vi "All Lamps OFF.vi"(7 "L1 Prime":bool=TRUE, 8 "error in (no error)":errorcluster) -> (0 "error out":T1)   [LabVIEW 2018]
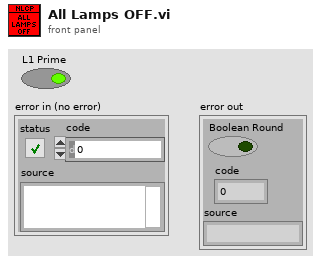
[diagram p1: front panel]
types:
  T1 = cluster{"Boolean Round":bool, "code":i32, "source":string}
  T2 = enum16{"Lamp A1", "Lamp B1", "Lamp C1", "Lamp D1", "Lamp E1", "Lamp F1", "Lamp G1", "Lamp H1", "Lamp A2", "Lamp B2", "Lamp C2", "Lamp D2", "Lamp E2", "Lamp F2", "Lamp G2", "Lamp H2", "Ack A1", "Ack B1", "Ack C1", "Ack D1", "Ack E1", "Ack F1", "Ack G1", "Ack H1", "Ack A2", "Ack B2", "Ack C2", "Ack D2", "Ack E2", "Ack F2", "Ack G2", "Ack H2", "SSM", "SAS", "LSM", ""}
  T3 = enum16{"Lamp A1", "Lamp B1", "Lamp C1", "Lamp D1", "Lamp E1", "Lamp F1", "Lamp G1", "Lamp H1", "Lamp A2", "Lamp B2", "Lamp C2", "Lamp D2", "Lamp E2", "Lamp F2", "Lamp G2", "Lamp H2", "Ack A1", "Ack B1", "Ack C1", "Ack D1", "Ack E1", "Ack F1", "Ack G1", "Ack H1", "Ack A2", "Ack B2", "Ack C2", "Ack D2", "Ack E2", "Ack F2", "Ack G2", "Ack H2", "SSM", "SAS", "LSM", ""}[]
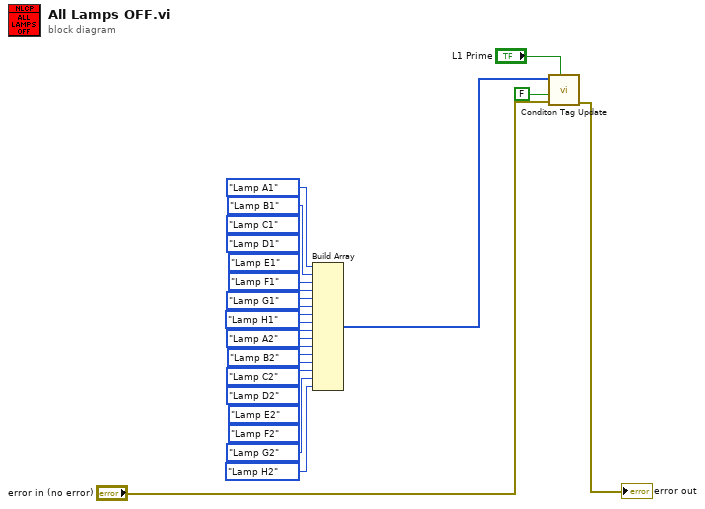
[diagram p0: block diagram]
diagram:
  n1 = Build Array(T2."Lamp A1" ("Tag"), T2."Lamp B1" ("Tag"), T2."Lamp C1" ("Tag"), T2."Lamp D1" ("Tag"), T2."Lamp E1" ("Tag"), T2."Lamp F1" ("Tag"), T2."Lamp G1" ("Tag"), T2."Lamp H1" ("Tag"), T2."Lamp A2" ("Tag"), T2."Lamp B2" ("Tag"), T2."Lamp C2" ("Tag"), T2."Lamp D2" ("Tag"), T2."Lamp E2" ("Tag"), T2."Lamp F2" ("Tag"), T2."Lamp G2" ("Tag"), T2."Lamp H2" ("Tag")) -> (w21:T3)
  n2 = call "Conditon Tag Update.vi"("L1 Prime"="L1 Prime", "error in (no error)"="error in (no error)", "OK?"=FALSE ("Boolean"), "Array"=w21) -> ("error out"=→"error out":T1)  [unwired: 7 in]
